vi "Log String Data.vi"(0 "Data Logger Interface in":refnum<class "Data Logger Actor Interface.lvclass">, 5 "Group Name (Untitled)":string, 7 "Channel Names (Untitled)":string[](array[string]), 9 "Data":string[][](array[string]), 11 "error in (no error)":errorcluster) -> (4 "Data Logger Interface out":refnum<class "Data Logger Actor Interface.lvclass">, 15 "error out":errorcluster)   [LabVIEW 2024, in "Data Logger Actor Interface.lvlib" / "Data Logger Actor Interface.lvclass"]
uses:
  Data Logger Actor Interface.lvclass
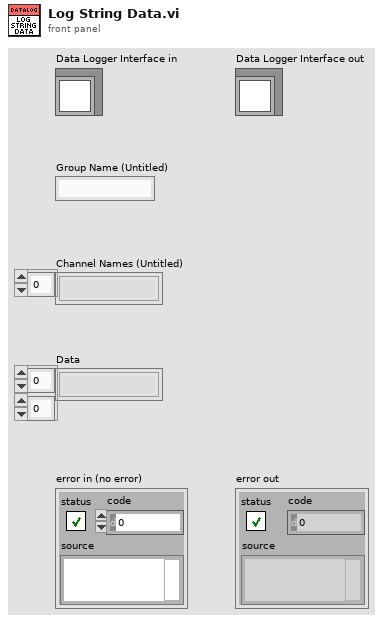
[diagram p1: front panel]
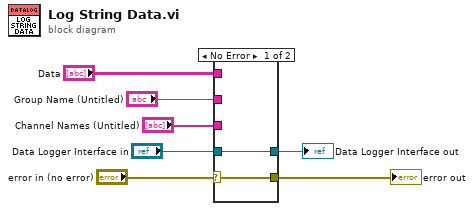
[diagram p0: block diagram]
diagram:
  n1 = case shown="No Error" "error in (no error)" {
    selector: "error in (no error)" -> [w8 w11]
    tunnel: [w8 w11] -> w6
    tunnel: [w9 w10] -> w4
    tunnel: "Data Logger Interface in" -> [w9 w10]
    tunnel: "Data" -> [_ _]
    tunnel: "Channel Names (Untitled)" -> [_ _]
    tunnel: "Group Name (Untitled)" -> [_ _]
    frame No Error {
    }
    frame Error {
    }
  }
  "error out" <- w6
  "Data Logger Interface out" <- w4
